vi "performaction.vi"(11 "command line arguments":T1) -> (0 "error out":errorcluster)   [LabVIEW 2018]
uses:
  executables/arguments.ctl
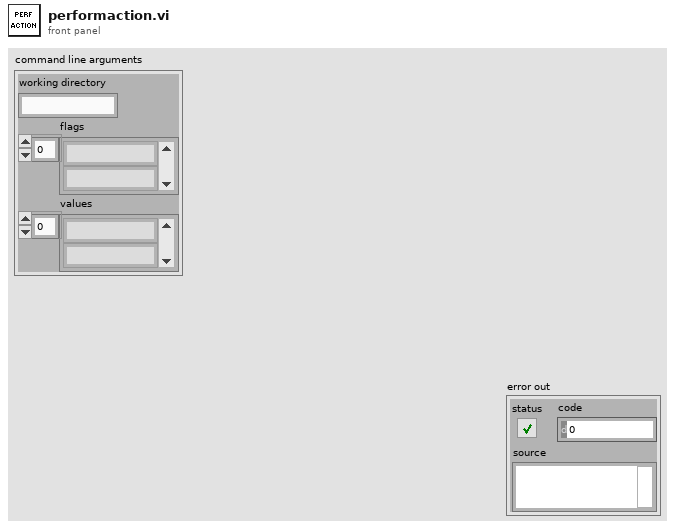
[diagram p1: front panel]
types:
  T1 = typedef "arguments.ctl" = cluster{"working directory":string, "flags":string[], "values":string[]}
  T2 = cluster{"working directory":string, "paths":string[], "args":string[]}
  T3 = cluster{"-noattr":bool, "-nofp":bool, "-nofppos":bool, "-nobd":bool, "-nobdcosm":bool, "-nobdpos":bool}
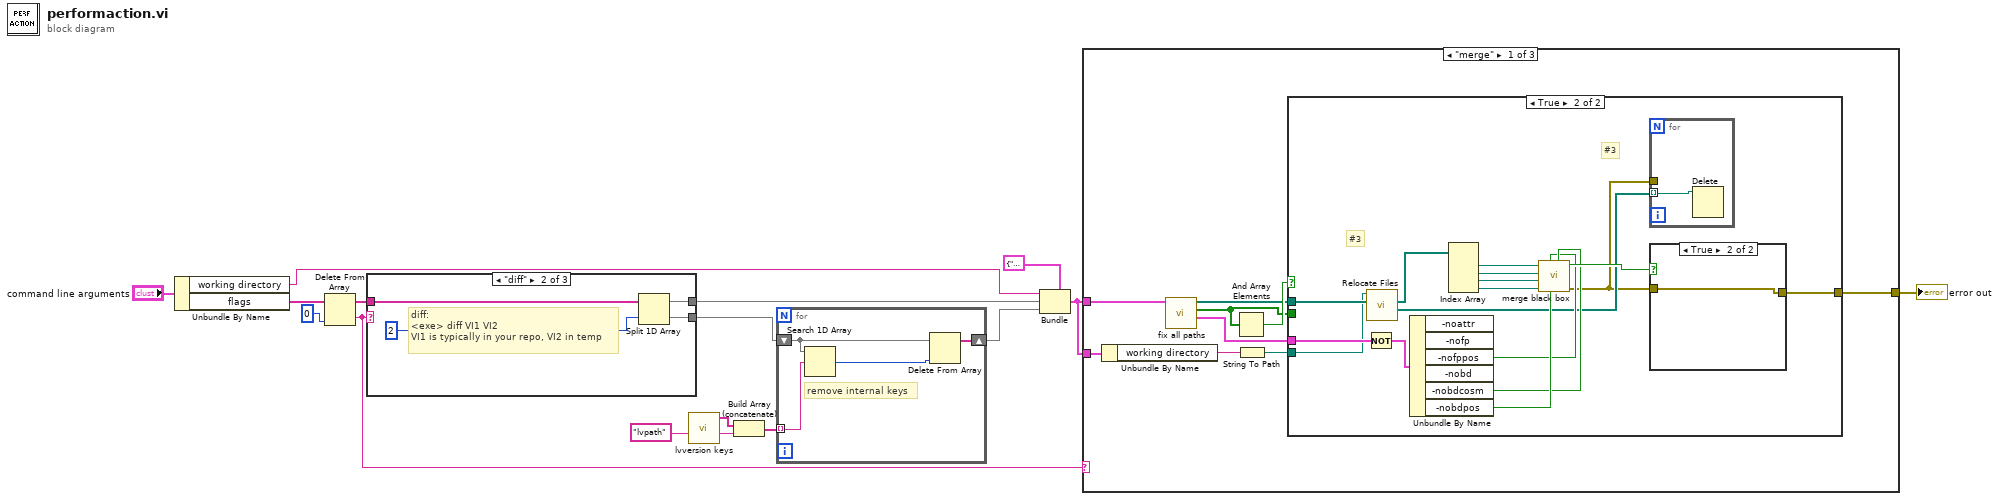
[diagram p0: block diagram]
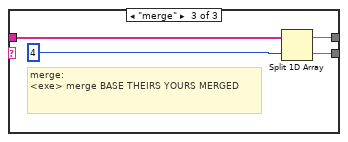
[diagram p3: hidden frame]
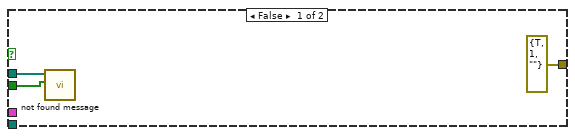
[diagram p4: hidden frame]
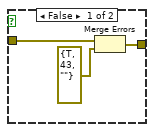
[diagram p5: hidden frame]
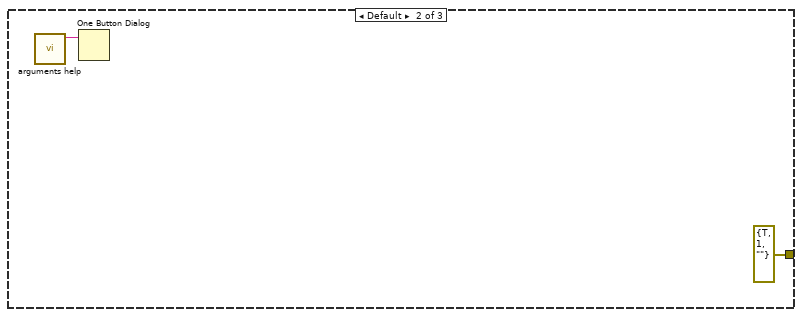
[diagram p6: hidden frame]
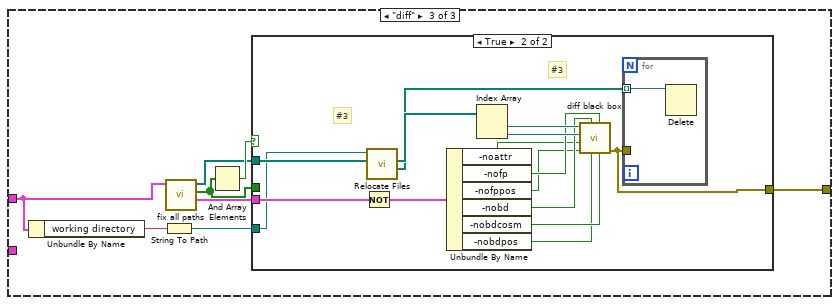
[diagram p7: hidden frame]
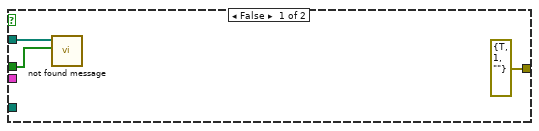
[diagram p8: hidden frame]
diagram:
  n1 = Unbundle By Name("command line arguments") -> ("working directory"=w8:string, "flags"=w12:string[])
  n2 = Delete From Array(array=w12, index=0) -> (deleted portion=w10:string, array with subset deleted=w9:string[])  [unwired: 1 in]
  n3 = case shown="\"diff\"" w10 {
    tunnel: w9 -> [w16 w20 w24]
    tunnel: [_ w18 w22] -> w7
    tunnel: [w16 w17 w21] -> w5
    frame Default {
    }
    frame "diff" {
      # "diff:\n<exe> diff VI1 VI2\nVI1 is typically in your repo, VI2 in temp"
      n4 = Split 1D Array(array=w20, index=2 ("length")) -> (first subarray=w18:string[], second subarray=w17:string[])
    }
    frame "merge" {
      # "merge:\n<exe> merge BASE THEIRS YOURS MERGED"
      n5 = Split 1D Array(array=w24, index=4 ("length")) -> (first subarray=w22:string[], second subarray=w21:string[])
    }
  }
  n6 = call "lvversion keys.vi"() -> ("lv version keys"=w13:string[])  [unwired: 11 in]
  n7 = Build Array (concatenate)(w13, "lvpath" ("String")) -> (w3:string[])
  n8 = for {
    shift-right: [w26] -> w4
    shift-left: w5 -> [w27]
    tunnel: w3 -> [w28] mode=indexing
    # "remove internal keys"
    n9 = Search 1D Array(1D array=w27, element=w28) -> (index of element=w25:i32)  [unwired: 1 in]
    n10 = Delete From Array(array=w27, index=w25) -> (array with subset deleted=w26:string[])  [unwired: 1 in, 1 out]
  }
  n11 = Bundle(cluster=T2 {"working directory"="", "paths"=[], "args"=[]} ("output cluster"), "working directory"=w8, "paths"=w7, "args"=w4) -> (w1:T2)
  n12 = case shown="\"merge\"" w10 {
    tunnel: [w34 errorcluster {"status"=TRUE, "code"=1, "source"=""} ("error out") w68] -> w15
    tunnel: w1 -> [w33 _ w66]
    tunnel: w1 -> [w31 _ _]
    frame "merge" {
      n13 = Unbundle By Name(w31) -> ("working directory"=w30:string)
      n14 = call "fix all paths.vi"("paths"=w33) -> ("settings"=w32:T3, "found"=w35:bool[], "paths out"=w36:path[])  [unwired: 8 in]
      n15 = And Array Elements(Boolean array=w35) -> (logical AND=w37:bool)
      n16 = String To Path(string=w30) -> (path=w29:path)
      n17 = case shown="True" w37 {
        tunnel: w36 -> [w40 w45]
        tunnel: w35 -> [w39 _]
        tunnel: [errorcluster {"status"=TRUE, "code"=1, "source"=""} ("error out") w51] -> w34
        tunnel: w32 -> [_ w50]
        tunnel: w29 -> [_ w41]
        frame False {
          n18 = call "not found message.vi"("found"=w39, "paths in"=w40) -> ()  [unwired: 10 in]
        }
        frame True {
          # "#3"
          # "#3"
          n19 = Not(x=w50) -> (.not. x?=w46:T3)
          n20 = call "Relocate Files.vi"("Paths in"=w45, "Working Folder"=w41) -> ("Files to delete"=w43:path[], "Paths out"=w44:path[])  [unwired: 8 in]
          n21 = Unbundle By Name(w46) -> ("-nofppos"=w47:bool, "-nobdcosm"=w48:bool, "-nobdpos"=w49:bool)  [unwired: 3 out]
          n22 = Index Array(array=w44) -> (element #1=w55:path, element #2=w54:path, element #3=w56:path, element #4=w53:path)  [unwired: 4 in]
          n23 = call "merge black box.vi"("BD Cosmetic?"=w48, "BD Pos/Size?"=w49, "FP Pos/Size?"=w47, "merge"=w53, "yours"=w56, "their"=w54, "base"=w55) -> ("error out"=w42:errorcluster, "Saved?"=w52:bool)  [unwired: 3 in]
          n24 = for {
            tunnel: w43 -> [w57] mode=indexing
            tunnel: w42 -> [_]
            n25 = Delete(path (use dialog)=w57) -> ()  [unwired: 4 in, 3 out]
          }
          n26 = case shown="True" w52 {
            tunnel: [w59 w61] -> w51
            tunnel: w42 -> [w60 w61]
            frame False {
              n27 = Merge Errors(w60, errorcluster {"status"=TRUE, "code"=43, "source"=""} ("error in")) -> (w59:errorcluster)
            }
            frame True {
            }
          }
        }
      }
    }
    frame Default {
      n28 = call "arguments help.vi"() -> ("args help"=w62:string)  [unwired: 11 in]
      n29 = One Button Dialog(message=w62) -> ()  [unwired: 1 in, 1 out]
    }
    frame "diff" {
      n30 = Unbundle By Name(w66) -> ("working directory"=w65:string)
      n31 = String To Path(string=w65) -> (path=w64:path)
      n32 = call "fix all paths.vi"("paths"=w66) -> ("settings"=w67:T3, "found"=w69:bool[], "paths out"=w70:path[])  [unwired: 8 in]
      n33 = And Array Elements(Boolean array=w69) -> (logical AND=w71:bool)
      n34 = case shown="True" w71 {
        tunnel: w70 -> [w74 w79]
        tunnel: w69 -> [w73 _]
        tunnel: [errorcluster {"status"=TRUE, "code"=1, "source"=""} ("error out") w75] -> w68
        tunnel: w67 -> [_ w87]
        tunnel: w64 -> [_ w77]
        frame False {
          n35 = call "not found message.vi"("found"=w73, "paths in"=w74) -> ()  [unwired: 10 in]
        }
        frame True {
          # "#3"
          # "#3"
          n36 = Not(x=w87) -> (.not. x?=w80:T3)
          n37 = call "Relocate Files.vi"("Paths in"=w79, "Working Folder"=w77) -> ("Files to delete"=w76:path[], "Paths out"=w78:path[])  [unwired: 8 in]
          n38 = Unbundle By Name(w80) -> ("-noattr"=w82:bool, "-nofp"=w84:bool, "-nofppos"=w81:bool, "-nobd"=w83:bool, "-nobdcosm"=w86:bool, "-nobdpos"=w85:bool)
          n39 = Index Array(array=w78) -> (element #1=w89:path, element #2=w88:path)  [unwired: 2 in]
          n40 = call "diff black box.vi"("BD Cosmetic?"=w86, "FP?"=w84, "BD Pos/Size?"=w85, "BD?"=w83, "FP Pos/Size?"=w81, "VI Attributes?"=w82, "VI2 Absolute"=w88, "VI1 Absolute"=w89) -> ("error out"=w75:errorcluster)  [unwired: 3 in]
          n41 = for {
            tunnel: w76 -> [w90] mode=indexing
            tunnel: w75 -> [_]
            n42 = Delete(path (use dialog)=w90) -> ()  [unwired: 4 in, 3 out]
          }
        }
      }
    }
  }
  "error out" <- w15
